vi "生成待输出D.vi"(11 "输出":T2) -> (3 "待输出操作":T1[](array[typedef]))   [LabVIEW 2017]
uses:
  Component Assemble Input.ctl
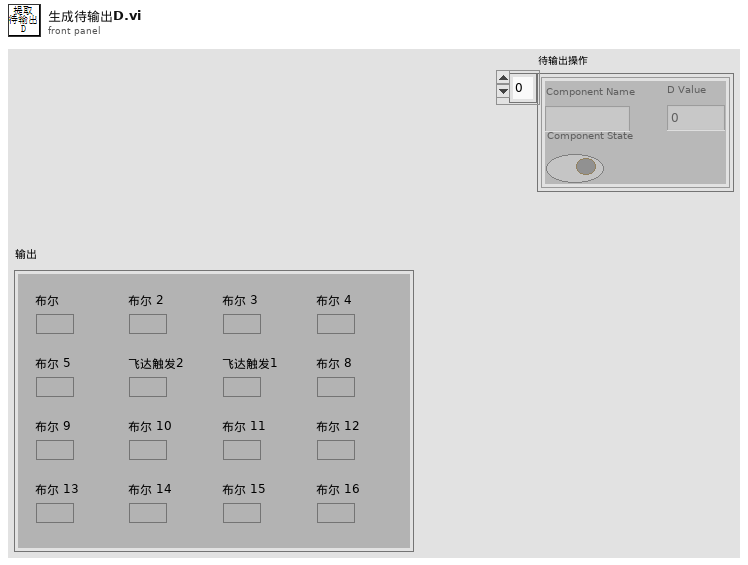
[diagram p1: front panel]
types:
  T1 = typedef "Component Assemble Input.ctl" = cluster{"Component Name":string, "Component State":bool, "D Value":i32}
  T2 = typedef "output控件.ctl" = cluster{"布尔":bool, "布尔 2":bool, "布尔 3":bool, "布尔 4":bool, "布尔 5":bool, "飞达触发2":bool, "飞达触发1":bool, "布尔 8":bool, "布尔 9":bool, "布尔 10":bool, "布尔 11":bool, "布尔 12":bool, "布尔 13":bool, "布尔 14":bool, "布尔 15":bool, "布尔 16":bool}
  T3 = typedef "配置检索操作.ctl" = enum16{"配置检索", "名称提取", "寄存器提取"}
  T4 = typedef "输入&输出配置提取集合.ctl" = cluster{"IO配置名称":string[], "IO配置点位地址":string[], "IO配置名称索引":i32[], "取反信息":i32[], "簇属性集合":string[]}
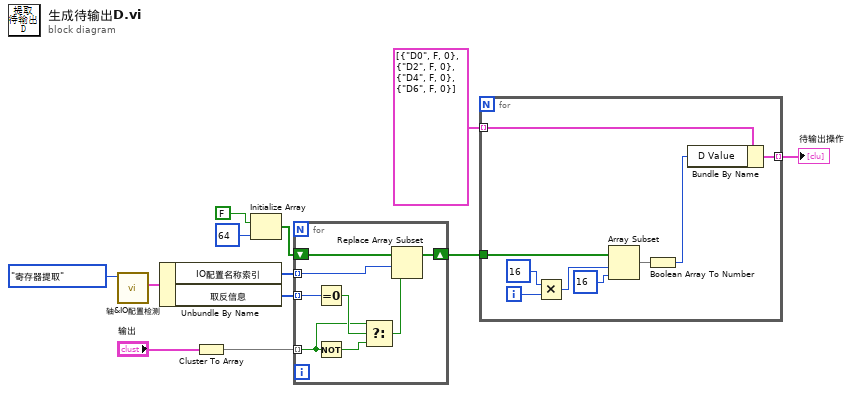
[diagram p0: block diagram]
diagram:
  n1 = call "轴&IO配置检测.vi"("配置检索操作"=配置检索操作."寄存器提取") -> ("输出配置提取集合"=w1:T4)  [unwired: 8 in, 2 out]
  n2 = Unbundle By Name(w1) -> ("IO配置名称索引"=w4:i32[], "取反信息"=w3:i32[])
  n3 = Cluster To Array(cluster="输出") -> (array=w5:bool[])
  n4 = Initialize Array(FALSE, 64 ("维数大小")) -> (w6:bool[])
  n5 = for {
    tunnel: w5 -> [w16] mode=indexing
    tunnel: w4 -> [w19] mode=indexing
    tunnel: w3 -> [w18] mode=indexing
    shift-right: [w13] -> w2
    shift-left: w6 -> [w20]
    n6 = Equal To 0?(x=w18) -> (x = 0?=w17:bool)
    n7 = Not(x=w16) -> (.not. x?=w15:bool)
    n8 = Select(t=w16, s=w17, f=w15) -> (s? t:f=w14:bool)
    n9 = Replace Array Subset(array=w20, new element=w14, index=w19) -> (w13:bool[])
  }
  n10 = for {
    tunnel: T1[] [{"Component Name"="D0", "Component State"=FALSE, "D Value"=0}, {"Component Name"="D2", "Component State"=FALSE, "D Value"=0}, {"Component Name"="D4", "Component State"=FALSE, "D Value"=0}, {"Component Name"="D6", "Component State"=FALSE, "D Value"=0}] -> [w25] mode=indexing
    tunnel: [w23] -> w8 mode=indexing
    tunnel: w2 -> [w22]
    i -> [w28]
    n11 = Multiply(x=16, y=w28) -> (x*y=w26:i32)
    n12 = Array Subset(array=w22, index=w26, length=16 ("长度")) -> (w21:bool[])
    n13 = Boolean Array To Number(Boolean array=w21) -> (number=w24:u32)
    n14 = Bundle By Name(cluster=w25, "D Value"=w24) -> (w23:T1)
  }
  "待输出操作" <- w8
